vi "TDMS2TDMInitializeLog.vi"(7 "Str Refnum":refnum<vi>, 8 "error in (no error)":errorcluster, 10 "TDM File Path":path, 11 "TDMS File Path":path) -> (0 "error out":errorcluster, 2 "TDM File Path Out":path, 3 "TDMS File Path Out":path)   [LabVIEW 2017]
doc: "This VI reads in the string control where the log text is stored. It also initializes the log with the names of the files to be converted and the date."
uses:
  <vilib>/Utility/tdmsutil.llb/TDMS2TDMLogOperation.ctl
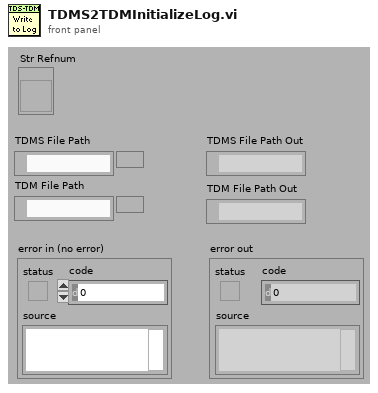
[diagram p1: front panel]
types:
  T1 = typedef "TDMS2TDMLogOperation.ctl" = enum16{"Initialize", "Data Conversion", "Name Conversion", "Write Log File"}
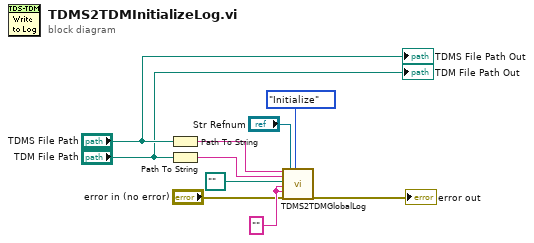
[diagram p0: block diagram]
diagram:
  w8 = "" ("Original Name")
  n1 = Path To String(path="TDMS File Path") -> (string=w4:string)
  n2 = Path To String(path="TDM File Path") -> (string=w3:string)
  n3 = call <vilib>:"TDMS2TDMGlobalLog.vi"("Original Name"=w4, "New Name"=w3, "Log File Path"=path "", "Original Datatype"=w8, "New Datatype"=w8, "error in (no error)"="error in (no error)", "Str Refnum"="Str Refnum", "Operation"=TDMS2TDMLogOperation."Initialize") -> ("error out"=→"error out":errorcluster)  [unwired: 11 in]
  "TDMS File Path Out" <- "TDMS File Path"
  "TDM File Path Out" <- "TDM File Path"
